vi "Single SSC Relay Fill Additional Error info.vi"(0 "SSC Relay in":T1, 11 "error in":errorcluster, 12 "previous error in":errorcluster) -> (4 "SSC Relay out":T1, 15 "error out":errorcluster)   [LabVIEW 2019]
doc: "This VI appends information to the error message from the SSC Relay cluster if an error is on error in, but not initial error.\n\nThis makes it easier to debug code as it provides the user which session/site/channel/pin actually threw the error."
uses:
  SSC Relay.ctl
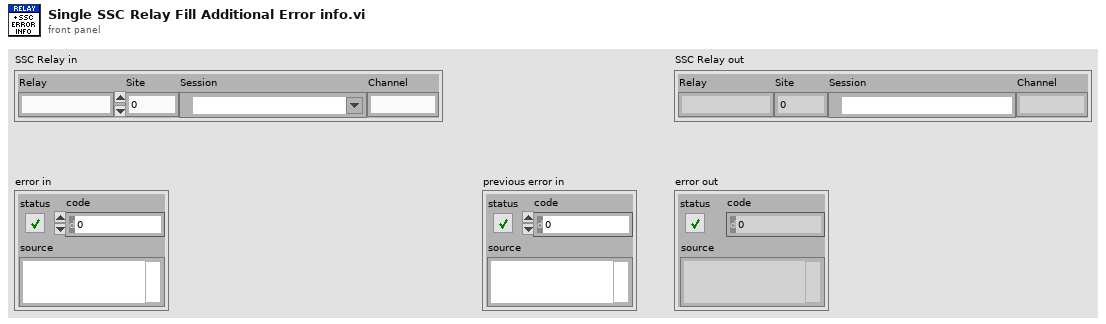
[diagram p1: front panel]
types:
  T1 = typedef "SSC Relay.ctl" = cluster{"Relay":string, "Site":i32, "Session":refnum<k15>, "Channel":string}
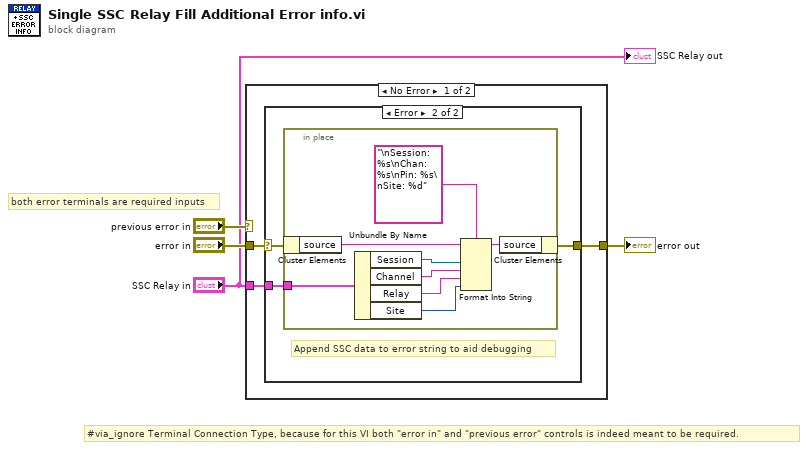
[diagram p0: block diagram]
diagram:
  # "#via_ignore Terminal Connection Type, because for this VI both \"error in\" and \"previous error\" controls is indeed meant to be required."
  # "both error terminals are required inputs"
  n1 = case shown="No Error" "previous error in" {
    selector: "previous error in" -> [_ w20]
    tunnel: [w6 w20] -> w3
    tunnel: "error in" -> [w7 _]
    tunnel: "SSC Relay in" -> [w5 _]
    frame No Error {
      n2 = case shown="Error" w7 {
        selector: w7 -> [w8 w11]
        tunnel: [w8 w9] -> w6
        tunnel: w5 -> [_ w10]
        frame No Error {
        }
        frame Error {
          # "Append SSC data to error string to aid debugging"
          n3 = in-place {
            in-place-border: w10 -> [w17]
            n4 = in-place-cluster #1(w11) -> ("source"=w19:string)
            n5 = Unbundle By Name(w17) -> ("Session"=w16:refnum<k15>, "Channel"=w15:string, "Relay"=w14:string, "Site"=w13:i32)
            n6 = Format Into String(format string="\nSession: %s\nChan: %s\nPin: %s\nSite: %d", initial string=w19, w16, w15, w14, w13) -> (resulting string=w18:string)  [unwired: 1 in, 1 out]
            n7 = in-place-cluster #1("source"=w18) -> (w9:errorcluster)
          }
        }
      }
    }
    frame Error {
      # "These errors already existed, leave them as they are"
    }
  }
  "error out" <- w3
  "SSC Relay out" <- "SSC Relay in"
